vi "Test Base Namer with extension with label.vi"   [LabVIEW 2020, in "Namer.Tests.lvclass"]
uses:
  Namer.Tests.lvclass
  Source/Approval Tests/Namer/Namer.lvclass
  Source/Approval Tests/Naming Data/Naming Data.lvclass
  Source/Approval Tests/Naming Data/Naming Data.lvclass/Naming Data.ctl
  Source/Approval Tests/Naming Data/Write Test VI Name.vi
  Source/Approval Tests/Naming Data/Write Extension.vi
  Source/Approval Tests/Naming Data/Write Test Label.vi
  <vilib>/addons/_JKI Toolkits/Caraya/classes/Assert/Assert Equal Value and Type_Variant.vi
  <vilib>/addons/_JKI Toolkits/Caraya/classes/Test/Test.lvclass
  <vilib>/addons/_JKI Toolkits/Caraya/classes/Assert/Assert.lvclass
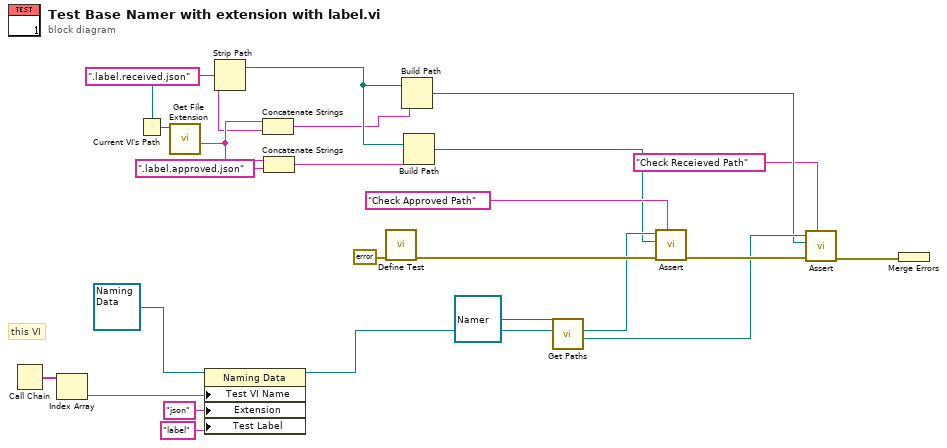
[diagram p0: block diagram]
diagram:
  # "this VI"
  n1 = Call Chain() -> (call chain=w19:string[])
  n2 = Index Array(array=w19) -> (element=w18:string)  [unwired: 1 in]
  n3 = Current VI's Path() -> (path=w12:path)
  n4 = call <vilib>:"Get File Extension.vi"("file"=w12) -> ("filename without extension"=w10:string)  [unwired: 6 in, 4 out]
  n5 = property on="Property Node" class="Naming Data"(reference=refnum<class "Naming Data.lvclass"> refnum ("Naming Data"), "Test VI Name"=w18, "Extension"="json", "Test Label"="label") -> (reference out=w17:refnum<class "Naming Data.lvclass">)  [unwired: 1 in, 1 out]
  n6 = Strip Path(path=w12) -> (stripped path=w11:path)  [unwired: 1 out]
  n7 = Concatenate Strings(w10, ".label.received.json" ("string")) -> (w7:string)
  n8 = Concatenate Strings(w10, ".label.approved.json" ("string")) -> (w6:string)
  n9 = call <vilib>:"Define Test.vi"("error in (no error)"=errorcluster {"status"=FALSE, "code"=0, "source"=""}) -> ("error out"=w23:errorcluster)  [unwired: 9 in, 1 out]
  n10 = Build Path(base path=w11, name or relative path=w7) -> (appended path=w5:path)
  n11 = Build Path(base path=w11, name or relative path=w6) -> (appended path=w4:path)
  n12 = call-dynamic "Get Paths.vi"("Naming Data"=w17, "Namer in"=refnum<class "Namer.lvclass"> refnum ("Approval Tests:Namer")) -> ("Received Path"=w13:path, "Approved Path"=w14:path)  [unwired: 6 in, 2 out]
  n13 = call-poly <vilib>:"Assert.vi"("Label"="Check Approved Path" ("Label (VI Title)"), "error in (no error)"=w23, "Y"=w4, "X"=w14) -> ("error out"=w16:errorcluster)  [unwired: 6 in, 1 out]
  n14 = call-poly <vilib>:"Assert.vi"("Label"="Check Receieved Path" ("Label (VI Title)"), "error in (no error)"=w16, "Y"=w5, "X"=w13) -> ("error out"=w15:errorcluster)  [unwired: 6 in, 1 out]
  n15 = Merge Errors(w15) -> ()  [unwired: 1 out]
